vi "generateEventHardpointActuatorInfo.vi"(8 "error in (no error)":errorcluster, 10 "EventHardpointActuatorInfo":T1, 11 "UserEvents in":refnum<class "UserEvents.lvclass">) -> (0 "error out":errorcluster, 3 "UserEvents out":refnum<class "UserEvents.lvclass">)   [LabVIEW 2016, in "UserEvents.lvclass"]
uses:
  UserEvents.lvclass
  DataTypes/Topics/EventHardpointActuatorInfo.ctl
  DataTypes/Topics/Parts/Timestamp.ctl
  UserEvents.lvclass/UserEvents.ctl
  DataTypes/Topics/M1M3SupportTopics.lvlib
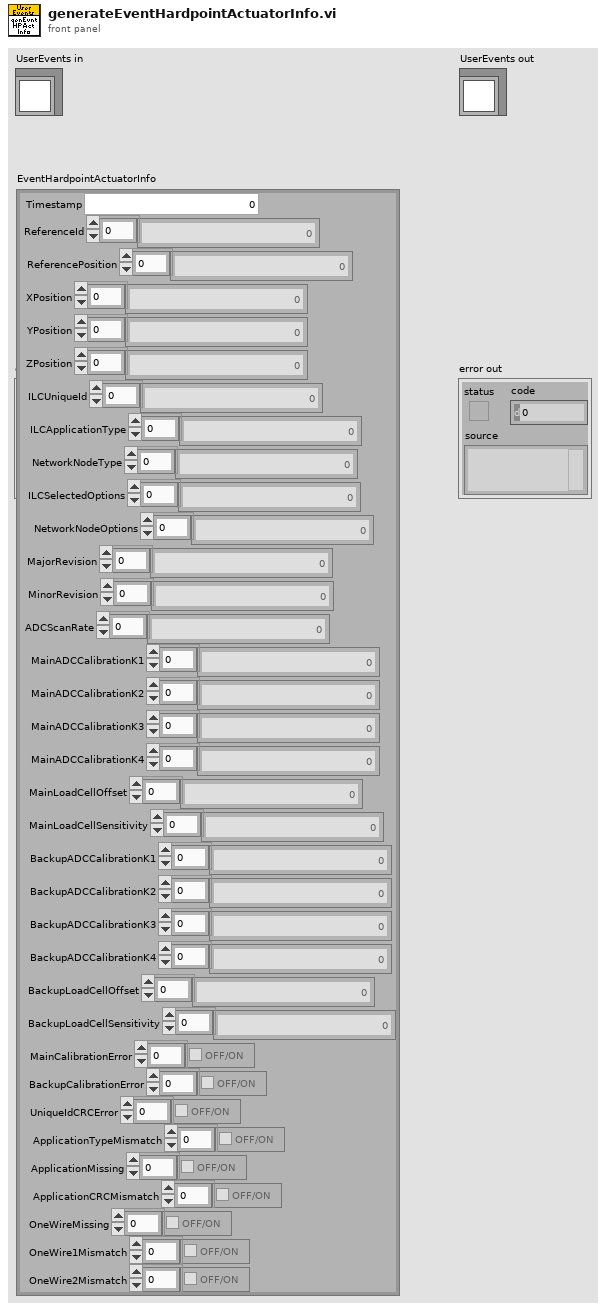
[diagram p1: front panel]
types:
  T1 = typedef "M1M3SupportTopics.lvlib/EventHardpointActuatorInfo.ctl" = cluster{"Timestamp":T2, "ReferenceId":i32[], "ReferencePosition":i32[], "XPosition":sgl[], "YPosition":sgl[], "ZPosition":sgl[], "ILCUniqueId":i64[], "ILCApplicationType":u8[], "NetworkNodeType":u8[], "ILCSelectedOptions":u8[], "NetworkNodeOptions":u8[], "MajorRevision":u8[], "MinorRevision":u8[], "ADCScanRate":u8[], "MainADCCalibrationK1":sgl[], "MainADCCalibrationK2":sgl[], "MainADCCalibrationK3":sgl[], "MainADCCalibrationK4":sgl[], "MainLoadCellOffset":sgl[], "MainLoadCellSensitivity":sgl[], "BackupADCCalibrationK1":sgl[], "BackupADCCalibrationK2":sgl[], "BackupADCCalibrationK3":sgl[], "BackupADCCalibrationK4":sgl[], "BackupLoadCellOffset":sgl[], "BackupLoadCellSensitivity":sgl[], "MainCalibrationError":bool[], "BackupCalibrationError":bool[], "UniqueIdCRCError":bool[], "ApplicationTypeMismatch":bool[], "ApplicationMissing":bool[], "ApplicationCRCMismatch":bool[], "OneWireMissing":bool[], "OneWire1Mismatch":bool[], "OneWire2Mismatch":bool[]}
  T2 = typedef "M1M3SupportTopics.lvlib/Timestamp.ctl" = dbl
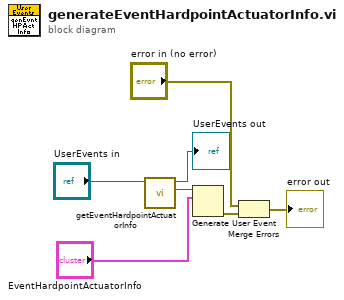
[diagram p0: block diagram]
diagram:
  n1 = call "getEventHardpointActuatorInfo.vi"("UserEvents in"="UserEvents in") -> ("EventHardpointActuatorInfo"=w7:refnum<user-event>, "UserEvents out"=→"UserEvents out":refnum<class "UserEvents.lvclass">)  [unwired: 9 in]
  n2 = Generate User Event(user event=w7, event data cluster="EventHardpointActuatorInfo") -> (error out=w3:errorcluster)  [unwired: 2 in, 1 out]
  n3 = Merge Errors("error in (no error)", w3) -> (→"error out":errorcluster)
